vi "search for Quanta Sonde devices.vi"(0 "VISA resource name":refnum<visa-resource-name>="COM13", 5 "Search for Comm Ports?":bool=TRUE, 11 "error in (no error)":errorcluster) -> (1 "Com Port with SDI-12 devices":refnum<visa-resource-name>[](array[refnum]), 3 "12V monitor":dbl, 4 "Com Port with Quanta Sonde devices":refnum<visa-resource-name>[](array[refnum]), 6 "Number of Quanta Sonde devices":i32, 10 "Number of Quanta Sonde devices > 0?":bool, 12 "Number of SDI-12 Devices":i32, 14 "H-4191 Adapter found":bool, 15 "Error Out":errorcluster)   [LabVIEW 2016]
panel:
  out "List of Com Ports Present in System":refnum<visa-resource-name>[](array[refnum])
  out "Number of Com Ports Present in System":i32
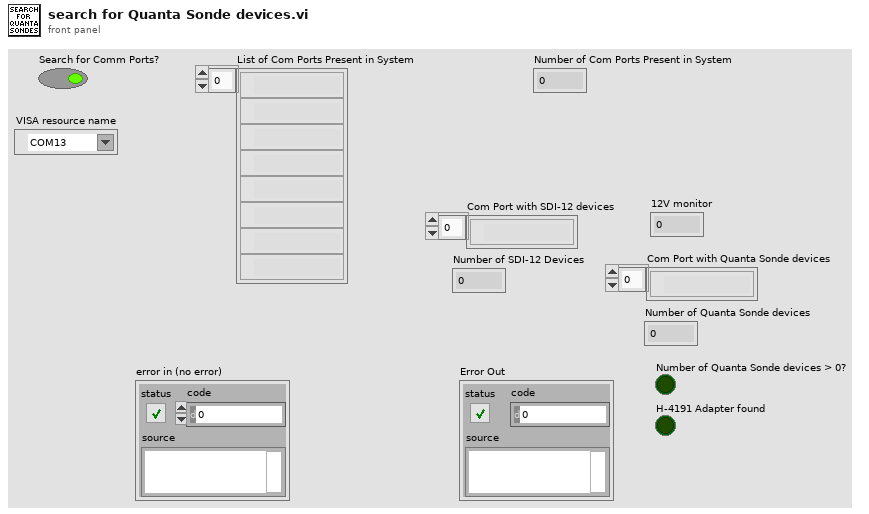
[diagram p1: front panel]
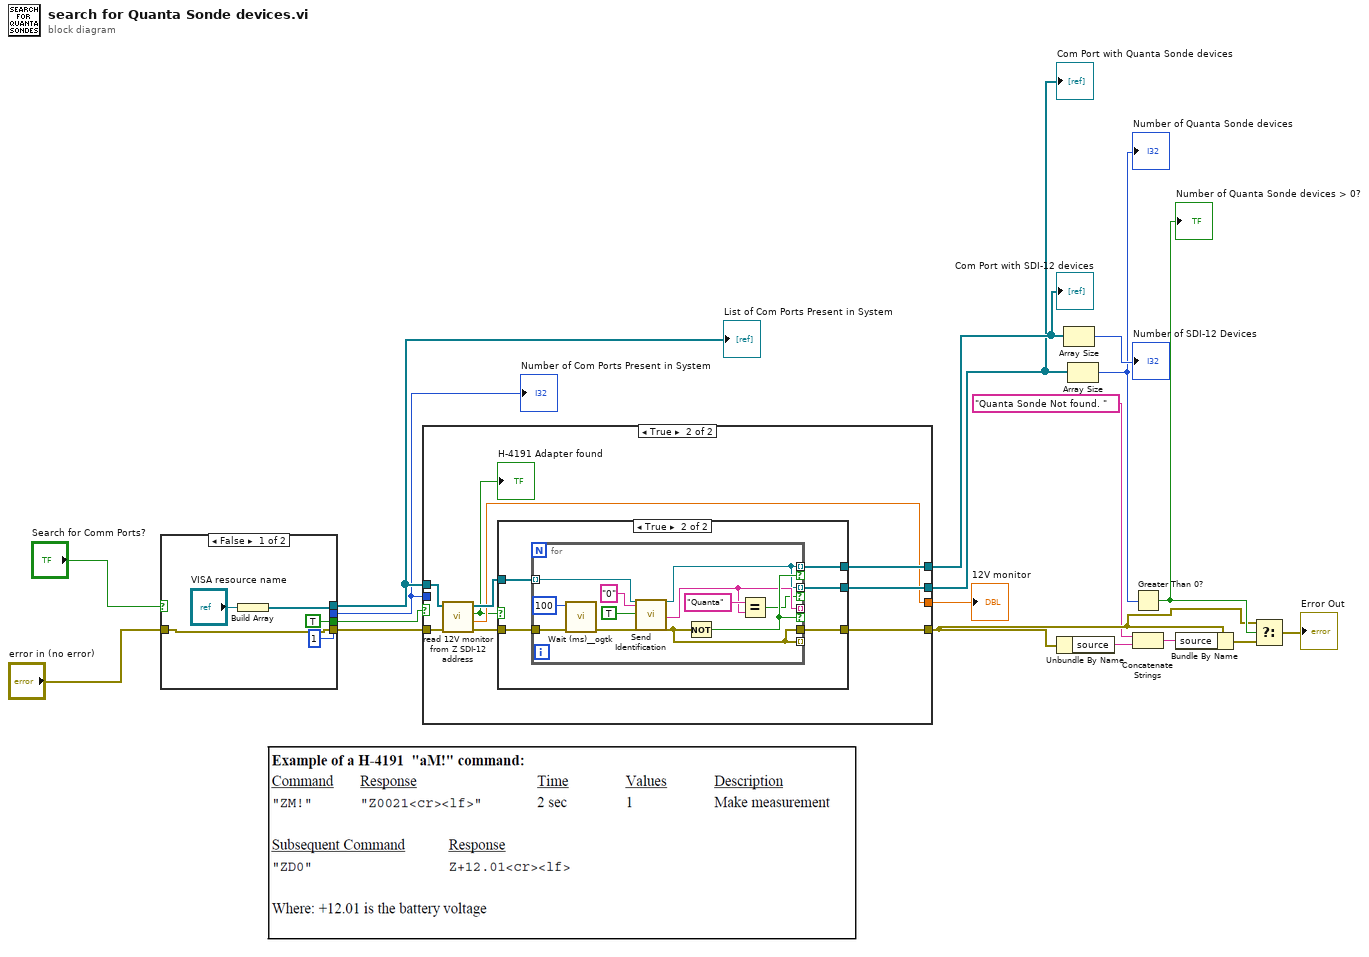
[diagram p0: block diagram]
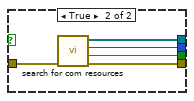
[diagram p2: hidden frame]
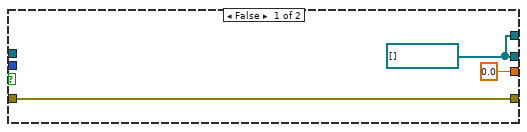
[diagram p3: hidden frame]
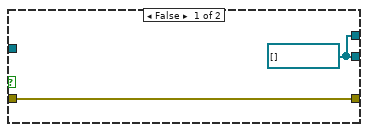
[diagram p4: hidden frame]
diagram:
  n1 = case shown="False" "Search for Comm Ports?" {
    tunnel: "error in (no error)" -> [w21 w28]
    tunnel: [TRUE ("Number of Com Ports Present in System > 0?") w27] -> w17
    tunnel: [w22 w26] -> w16
    tunnel: [w21 w25] -> w15
    tunnel: [1 ("Number of Com Ports Present in System") w24] -> w10
    frame False {
      n2 = Build Array("VISA resource name") -> (w22:refnum<visa-resource-name>[])
    }
    frame True {
      n3 = call "search for com resources.vi"("error in (no error)"=w28) -> ("error out"=w25:errorcluster, "Number of Com Ports Present in System > 0?"=w27:bool, "Number of Com Ports Present in System"=w24:i32, "List of Com Ports Present in System"=w26:refnum<visa-resource-name>[])  [unwired: 7 in]
    }
  }
  "Number of Com Ports Present in System" <- w10
  "List of Com Ports Present in System" <- w16
  n4 = case shown="True" w17 {
    tunnel: w16 -> [_ w37]
    tunnel: w15 -> [w31 w36]
    tunnel: [w30 w40] -> w14
    tunnel: [w31 w39] -> w5
    tunnel: [w30 w38] -> w12
    tunnel: w10 -> [_ _]
    tunnel: [0.0 ("12V monitor") w33] -> w9
    frame False {
      w30 = refnum<visa-resource-name>[] []
    }
    frame True {
      n5 = call "read 12V monitor from Z SDI-12 address.vi"("error in (no error)"=w36, "List of Com Ports Present in System"=w37) -> ("error out"=w35:errorcluster, "12V monitor"=w33:dbl, "H-4191 Adapter found"=w32:bool, "List of Com Ports Present in System 2"=w34:refnum<visa-resource-name>[])  [unwired: 6 in]
      "H-4191 Adapter found" <- w32
      n6 = case shown="True" w32 {
        tunnel: [w42 w47] -> w40
        tunnel: [w41 w46] -> w39
        tunnel: [w42 w45] -> w38
        tunnel: w35 -> [w41 w44]
        tunnel: w34 -> [_ w43]
        frame False {
          w42 = refnum<visa-resource-name>[] []
        }
        frame True {
          n7 = for {
            tunnel: w43 -> [w57] mode=indexing
            tunnel: w44 -> [w59]
            tunnel: [w51] -> w47 mode=indexing if=w54
            tunnel: [w55] -> _ mode=indexing
            tunnel: [w55] -> w46
            tunnel: [w52] -> _ mode=indexing if=w54
            tunnel: [w51] -> w45 mode=indexing if=w50
            n8 = call <userlib>:"Wait (ms)__ogtk.vi"("error in (no error)"=w59, "milliseconds to wait"=u32 100) -> ("error out"=w49:errorcluster)  [unwired: 8 in, 1 out]
            n9 = call "Send Identification.vi"("RS232 Port In"=w57, "Sensor Address In"="0", "Initialize/Close?"=TRUE, "Error In (No Error)"=w49) -> ("RS232 Port Out"=w51:refnum<visa-resource-name>, "Sensor Model Number"=w52:string, "Error Out"=w55:errorcluster)  [unwired: 16 in, 5 out]
            n10 = Not(x=w55) -> (.not. x?=w54:bool)
            n11 = Equal?(x="Quanta" ("Sensor Model Number"), y=w52) -> (x = y?=w50:bool)
          }
        }
      }
    }
  }
  "Com Port with SDI-12 devices" <- w14
  "Com Port with Quanta Sonde devices" <- w12
  "12V monitor" <- w9
  n12 = Unbundle By Name(w5) -> ("source"=w4:string)
  n13 = Array Size(array=w14) -> (size(s)=→"Number of SDI-12 Devices":i32)
  n14 = Array Size(array=w12) -> (size(s)=w11:i32)
  "Number of Quanta Sonde devices" <- w11
  n15 = Greater Than 0?(x=w11) -> (x > 0?=w7:bool)
  "Number of Quanta Sonde devices > 0?" <- w7
  n16 = Concatenate Strings("Quanta Sonde Not found. " ("source"), w4) -> (w3:string)
  n17 = Bundle By Name(cluster=w5, "source"=w3) -> (w6:errorcluster)
  n18 = Select(t=w5, s=w7, f=w6) -> (s? t:f=→"Error Out":errorcluster)
